vi "LibXML_AddChild.vi"(8 "error in":errorcluster, 10 "parent":u32, 11 "node":u32) -> (0 "error out":errorcluster, 3 "node copy":u32)   [LabVIEW 2019, in "Tools.lvlib" / "LibXML.lvlib"]
doc: "libXML2:\nxmlNodePtr xmlAddChild (xmlNodePtr parent, xmlNodePtr cur)\n\nAdd a new node to @parent, at the end of the child (or property) list merging adjacent TEXT nodes\n(in which case @cur is freed) If the new node is ATTRIBUTE, it is added into properties instead of children.\nIf there is an attribute with equal name, it is first destroyed.\n\nparent: the parent node\ncur: the child node\nReturns: the child or NULL in case of error."
uses:
  LibXML.lvlib
  dll/libxml2.dll
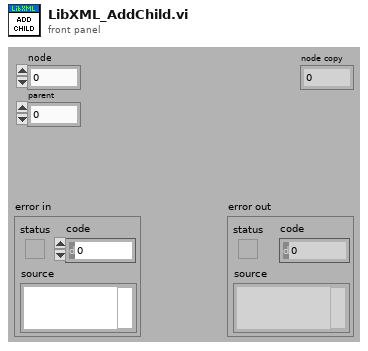
[diagram p1: front panel]
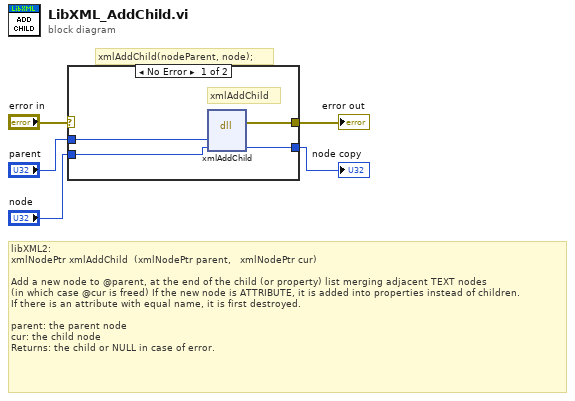
[diagram p0: block diagram]
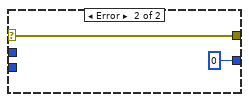
[diagram p2: hidden frame]
diagram:
  # "libXML2:\nxmlNodePtr\txmlAddChild\t\t(xmlNodePtr parent, \t xmlNodePtr cur)\n\nAdd a new node to @parent, at the end of the child (or property) list merging adjacent TEXT nodes\n(in which case @cur is freed) If the new node is ATTRIBUTE, it is added into properties instead of children.\nIf there is an attribute with equal name, it is first destroyed.\n\nparent:\tthe parent node\ncur:\tthe child node\nReturns:\tthe child or NULL in case of error."
  # "xmlAddChild(nodeParent, node);"
  n1 = case shown="No Error" "error in" {
    selector: "error in" -> [_ w11]
    tunnel: [w9 w11] -> w4
    tunnel: "parent" -> [w8 _]
    tunnel: "node" -> [w7 _]
    tunnel: [w6 u32 0 ("node")] -> w1
    frame No Error {
      # "xmlAddChild"
      n2 = dll-call lib="C:/Projects/_Prywatne/MyCIT/Framework/Tools/XML/LibXML/dll/libxml2.dll" fn="xmlAddChild"("parent"=w8, "node"=w7) -> (error out=w9:errorcluster, "node"=w6:u32)  [unwired: 5 in, 1 out]
    }
    frame Error {
    }
  }
  "error out" <- w4
  "node copy" <- w1
